vi "Read Window Title.vi"(8 "error in (no error)":errorcluster, 11 "MGI_Progress Bar Options In":refnum<class "Progress Bar Settings.lvclass">) -> (0 "error out":errorcluster, 2 "Window Title":string="Progress", 3 "MGI_Progress Bar Options Out":refnum<class "Progress Bar Settings.lvclass">)   [LabVIEW 2016, in "Progress Bar Settings.lvclass"]
uses:
  <userlib>/_MGI/User Interface/Progress Bar/Progress Bar Settings/Progress Bar Settings.lvclass
  <userlib>/_MGI/User Interface/Progress Bar/Progress Bar Settings/Progress Bar Settings.lvclass/Progress Bar Settings.ctl
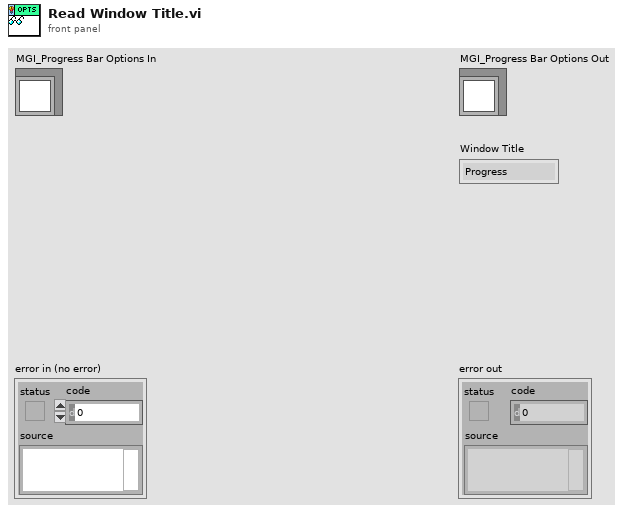
[diagram p1: front panel]
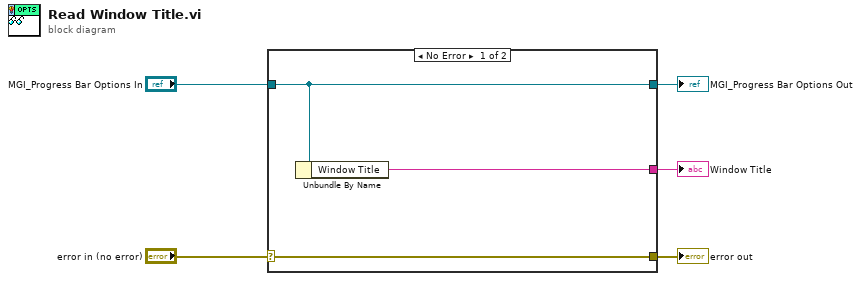
[diagram p0: block diagram]
diagram:
  n1 = case shown="No Error" "error in (no error)" {
    selector: "error in (no error)" -> [w8 w9]
    tunnel: [w8 w9] -> w4
    tunnel: [w7 w10] -> w2
    tunnel: "MGI_Progress Bar Options In" -> [w7 w10]
    tunnel: [w6 _] -> w1
    frame No Error {
      n2 = Unbundle By Name(w7) -> ("Window Title"=w6:string)
    }
    frame Error {
    }
  }
  "error out" <- w4
  "MGI_Progress Bar Options Out" <- w2
  "Window Title" <- w1
